vi "MakeDataFileForMultiplot_MATLAB.vi"(0 "Desired Legends":string[](array[string]), 1 "1D Folder":path, 3 "Plot Array":cluster{"Angle":dbl[], "Radius":dbl[]}[](array[cluster]), 5 "xAxisBounds":T1={"Min"={"Auto"=TRUE, "Value"=0.0}, "Max"={"Auto"=TRUE, "Value"=0.0}}, 7 "yAxisBounds":T1={"Min"={"Auto"=TRUE, "Value"=0.0}, "Max"={"Auto"=TRUE, "Value"=0.0}}, 9 "Interation number":i32, 11 "Plot Number":i32, 13 "Error Bar Type":T3=enum."Standard Error") -> (2 "Data Directories":string[](array[string]), 4 "Plot Array":i32[](array[numeric]), 6 "X Label":string, 8 "Max Min array":dbl[][](array[numeric]), 10 "Error Bars":bool[](array[boolean]), 12 "File String":string, 14 "Y Label":string, 15 "Plot Number 2":i32)   [LabVIEW 2021]
uses:
  Anemometry/Anemometry Sub Vis/Data_plotting_vis/Results_plotter_Global.vi
  Anemometry/Anemometry Sub Vis/Data_plotting_vis/Error bar Type.ctl
  Anemometry/Anemometry Sub Vis/Data_plotting_vis/gnuplotScriptComponents/AutoManualNumber.ctl
  Anemometry/Anemometry Sub Vis/Data_plotting_vis/gnuplotScriptComponents/minAndMax.ctl
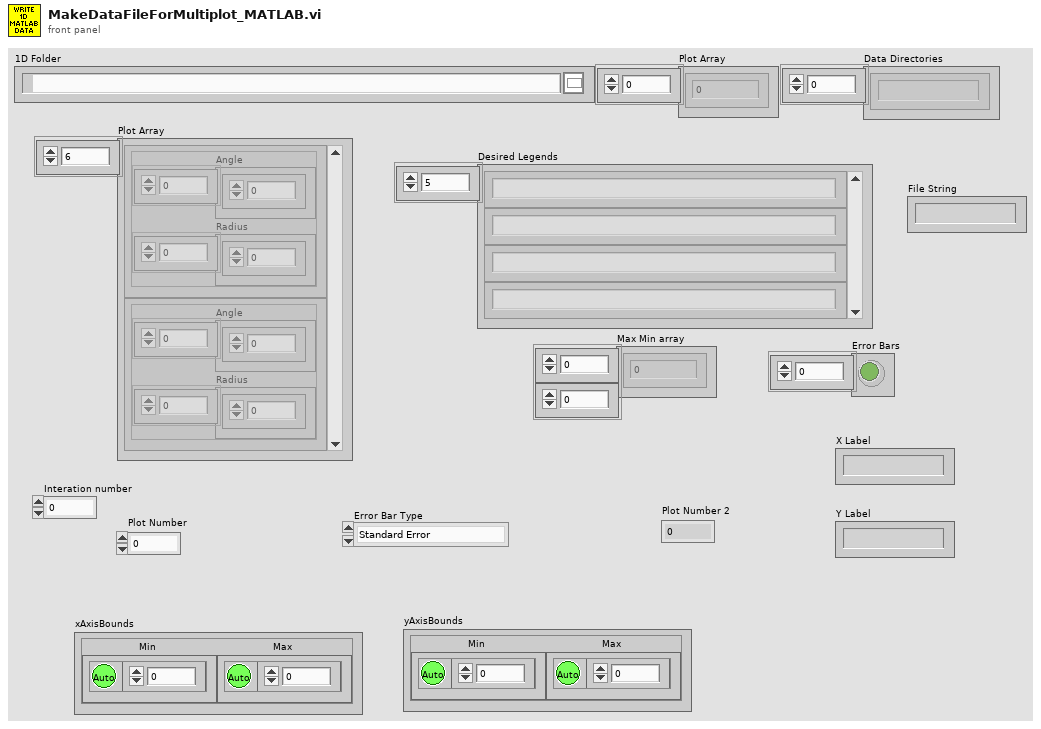
[diagram p1: front panel]
types:
  T1 = typedef "minAndMax.ctl" = cluster{"Min":T2, "Max":T2}
  T2 = typedef "AutoManualNumber.ctl" = cluster{"Auto":bool, "Value":dbl}
  T3 = typedef "Error bar Type.ctl" = enum16{"None", "Standard Error", "Separate upper and lower"}
  T4 = typedef "RFP_Plot_Metadata.ctl" = cluster{"Row Number":i32[], "Error Bars":T5, "X Label":string, "Y Label":string, "Blanks NaNs":i32[]}
  T5 = typedef "Error_bars_index.ctl" = cluster{"Upper":i32, "Lower":i32, "St Error":i32}
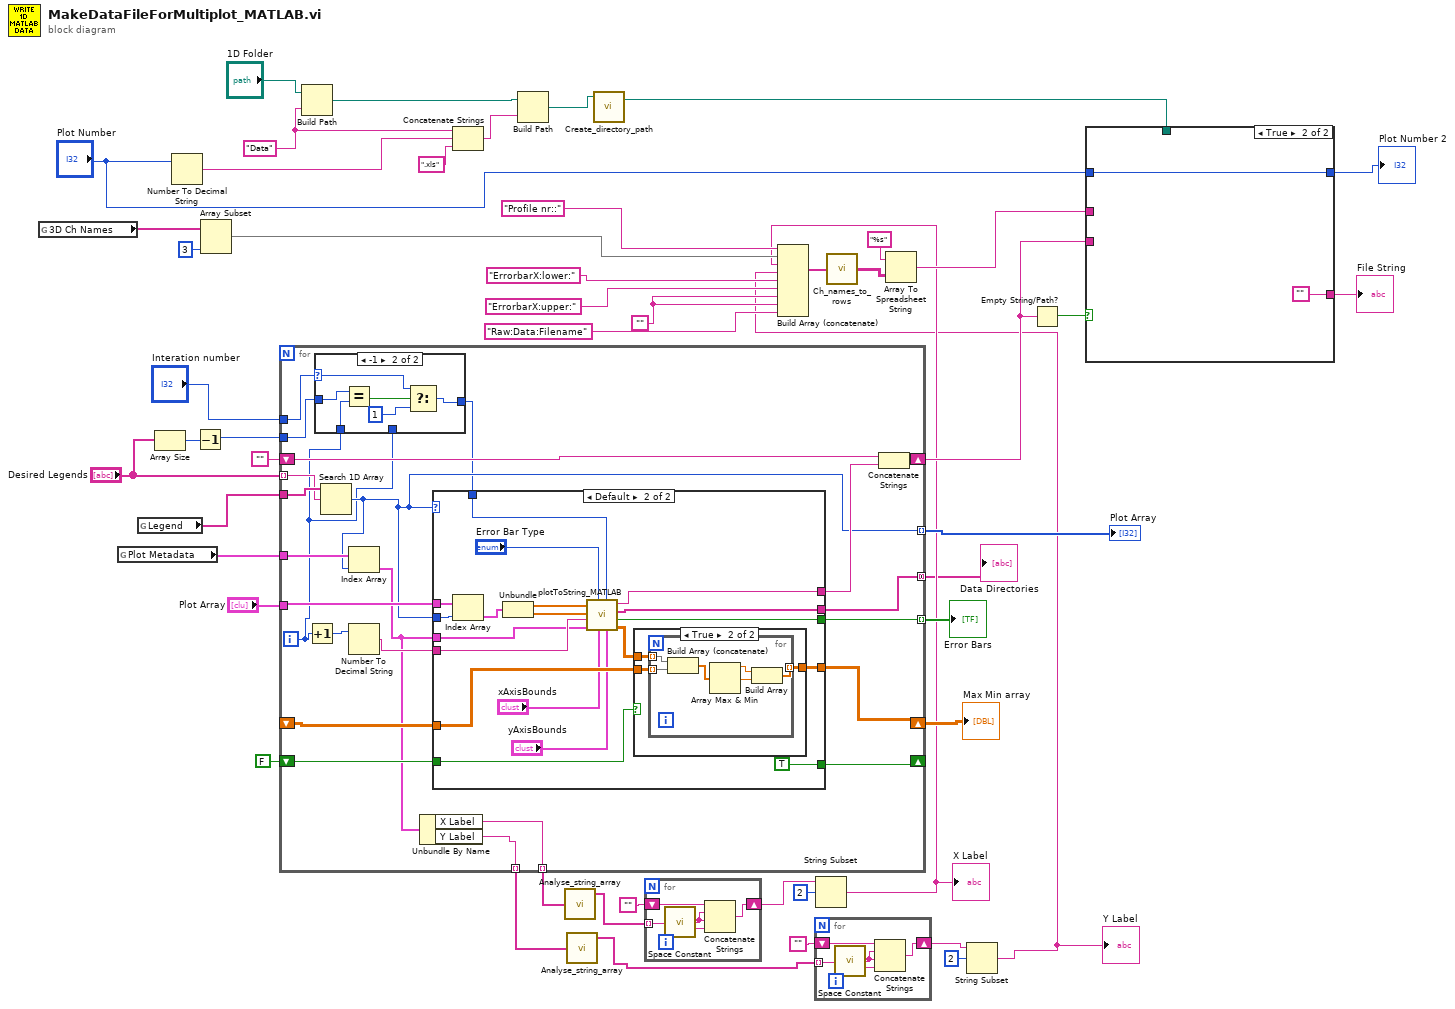
[diagram p0: block diagram]
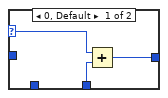
[diagram p2: hidden frame]
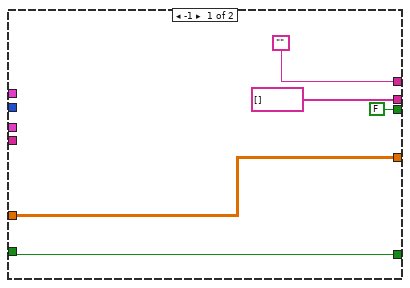
[diagram p3: hidden frame]
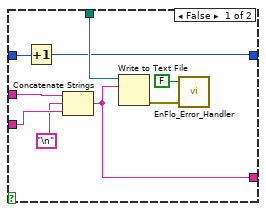
[diagram p5: hidden frame]
diagram:
  w31 = ""
  w50 = "Data" ("string")
  n1 = global read "Results_plotter_Global.vi" "3D Ch Names"() -> (w30:string[])
  n2 = global read "Results_plotter_Global.vi" "Plot Metadata"() -> (w19:T4[])
  n3 = global read "Results_plotter_Global.vi" "Legend"() -> (w26:string[])
  n4 = Array Size(array="Desired Legends") -> (size(s)=w2:i32)
  n5 = Number To Decimal String(number="Plot Number") -> (decimal integer string=w36:string)  [unwired: 1 in]
  n6 = Decrement(x=w2) -> (x-1=w1:i32)
  n7 = Array Subset(array=w30, length=3) -> (w28:string[])  [unwired: 1 in]
  n8 = for {
    tunnel: "Plot Array" -> [w69]
    shift-right: [w73] -> w22
    shift-left: "" -> [w72]
    tunnel: "Desired Legends" -> [w66] mode=indexing
    tunnel: w26 -> [w71]
    tunnel: [w59] -> w21 mode=indexing
    shift-right: [w65] -> w24
    shift-left: _ -> [w62]
    shift-right: [w63] -> _
    shift-left: FALSE -> [w64]
    tunnel: [w61] -> w20 mode=indexing
    tunnel: w19 -> [w60]
    tunnel: [w57] -> w18 mode=indexing
    tunnel: [w56] -> w17 mode=indexing
    tunnel: [w55] -> w6 mode=concatenating
    tunnel: "Interation number" -> [w54]
    tunnel: w1 -> [w51]
    i -> [w52]
    n9 = Increment(x=w52) -> (x+1=w68:i32)
    n10 = case shown="-1" w54 {
      selector: w54 -> [w75 w78]
      tunnel: w52 -> [w76 _]
      tunnel: [w74 w80] -> w53
      tunnel: w52 -> [_ w82]
      tunnel: w51 -> [_ w81]
      frame 0, Default {
        n11 = Add(x=w75, y=w76) -> (x+y=w74:i32)
      }
      frame -1 {
        n12 = Equal?(x=w81, y=w82) -> (x = y?=w79:bool)
        n13 = Select(t=w78, s=w79, f=1) -> (s? t:f=w80:i32)
      }
    }
    n14 = Search 1D Array(1D array=w71, element=w66) -> (index of element=w59:i32)  [unwired: 1 in]
    n15 = Index Array(array=w60, index=w59) -> (element=w58:T4)
    n16 = Number To Decimal String(number=w68) -> (decimal integer string=w67:string)  [unwired: 1 in]
    n17 = Unbundle By Name(w58) -> ("X Label"=w57:string, "Y Label"=w56:string)
    n18 = case shown="Default" w59 {
      tunnel: ["" w104] -> w70
      tunnel: w59 -> [_ w103]
      tunnel: w69 -> [_ w102]
      tunnel: w67 -> [_ w100]
      tunnel: [w85 w98] -> w65
      tunnel: w64 -> [w86 w96]
      tunnel: [w86 TRUE] -> w63
      tunnel: w62 -> [w85 w94]
      tunnel: [FALSE ("Error Bars?") w93] -> w61
      tunnel: w58 -> [_ w92]
      tunnel: [string[] [] ("Data Directories") w89] -> w55
      tunnel: w53 -> [_ w88]
      frame -1 {
      }
      frame Default {
        n19 = Index Array(array=w102, index=w103) -> (element=w101:cluster{"Angle":dbl[], "Radius":dbl[]})
        n20 = Unbundle(w101) -> ("Angle"=w105:dbl[], "Radius"=w106:dbl[])
        n21 = call "plotToString_MATLAB.vi"("yAxisBounds"="yAxisBounds", "Interation number"=w88, "xAxisBounds"="xAxisBounds", "Error Bar Type"="Error Bar Type", "Plot Metadata"=w92, "Profile Number"=w100, "Column2"=w106, "Column1"=w105) -> ("Max Min array"=w97:dbl[][], "Error Bars?"=w93:bool, "Data Directories"=w89:string[], "plotString"=w104:string)
        n22 = case shown="True" w96 {
          tunnel: [w107 w108] -> w98
          tunnel: w97 -> [w107 w110]
          tunnel: w94 -> [_ w109]
          frame False {
          }
          frame True {
            n23 = for {
              tunnel: w110 -> [w116] mode=indexing
              tunnel: w109 -> [w115] mode=indexing
              tunnel: [w111] -> w108 mode=indexing
              n24 = Build Array (concatenate)(w116, w115) -> (w114:dbl[])
              n25 = Array Max & Min(array=w114) -> (max value=w113:dbl, min value=w112:dbl)  [unwired: 2 out]
              n26 = Build Array(w113, w112) -> (w111:dbl[])
            }
          }
        }
      }
    }
    n27 = Concatenate Strings(w72, w70) -> (w73:string)
  }
  "Plot Array" <- w21
  "Max Min array" <- w24
  "Error Bars" <- w20
  "Data Directories" <- w6
  n28 = Build Path(base path="1D Folder", name or relative path=w50) -> (appended path=w48:path)
  n29 = Concatenate Strings(w50, w36, ".xls" ("string")) -> (w49:string)
  n30 = Build Path(base path=w48, name or relative path=w49) -> (appended path=w47:path)
  n31 = call "Analyse_string_array.vi"("String array"=w18) -> ("Unique strings"=w16:string[])  [unwired: 1 in, 1 out]
  n32 = call "Analyse_string_array.vi"("String array"=w17) -> ("Unique strings"=w13:string[])  [unwired: 1 in, 1 out]
  n33 = call "Create_directory_path.vi"("Path name"=w47) -> ("Path name Out"=w46:path)  [unwired: 2 in, 1 out]
  n34 = for {
    shift-right: [w117] -> w12
    shift-left: "" -> [w120]
    tunnel: w16 -> [w118] mode=indexing
    n35 = call <vilib>:"Space Constant.vi"() -> ("String"=w119:string)
    n36 = Concatenate Strings(w120, w119, w119, w118) -> (w117:string)
  }
  n37 = for {
    shift-right: [w121] -> w8
    shift-left: "" -> [w124]
    tunnel: w13 -> [w122] mode=indexing
    n38 = call <vilib>:"Space Constant.vi"() -> ("String"=w123:string)
    n39 = Concatenate Strings(w124, w123, w123, w122) -> (w121:string)
  }
  n40 = String Subset(string=w12, offset (0)=2) -> (substring=w10:string)  [unwired: 1 in]
  "X Label" <- w10
  n41 = String Subset(string=w8, offset (0)=2) -> (substring=w7:string)  [unwired: 1 in]
  "Y Label" <- w7
  n42 = Build Array (concatenate)("Profile nr::", w28, w10, w7, "ErrorbarX:lower:", "ErrorbarX:upper:", w31, w31, "Raw:Data:Filename" ("element")) -> (w42:string[])
  n43 = call "Ch_names_to_rows.vi"("Channel Names"=w42) -> ("3 Row names"=w40:string[][])
  n44 = Array To Spreadsheet String(array=w40, 3:"%s" ("format string")) -> (spreadsheet string=w39:string)  [unwired: 1 out]
  n45 = Empty String/Path?(string/path=w22) -> (empty?=w35:bool)
  n46 = case shown="True" w35 {
    tunnel: w46 -> [w133 _]
    tunnel: w39 -> [w132 _]
    tunnel: w22 -> [w127 _]
    tunnel: [w128 w135] -> w34
    tunnel: "Plot Number" -> [w129 w135]
    tunnel: [w125 ""] -> w5
    frame False {
      n47 = Increment(x=w129) -> (x+1=w128:i32)
      n48 = Concatenate Strings(w132, "\n", w127) -> (w125:string)
      n49 = Write to Text File(file (use dialog)=w133, text=w125) -> (error out=w131:errorcluster)  [unwired: 2 in, 2 out]
      n50 = call "EnFlo_Error_Handler.vi"("error in (no error)"=w131, "Dialog Box (F)"=FALSE ("Dialog Box (T)")) -> ()  [unwired: 2 in, 2 out]
    }
    frame True {
    }
  }
  "Plot Number 2" <- w34
  "File String" <- w5
